vi "ReadTiffPage_next.vi"(0 "TIFF file":T2 {"BigTiff,Endian" items=["Big-Endian"=0, "Native"=1, "Little-Endian"=2, "BigTiff-Big-Endian"=256, "Bigtiff,Native"=257, "Biftiff,Littleendian"=258]}, 2 "IFDoffset":i64, 3 "error in":errorcluster) -> (6 "TIFF file out":T2 {"BigTiff,Endian" items=["Big-Endian"=0, "Native"=1, "Little-Endian"=2, "BigTiff-Big-Endian"=256, "Bigtiff,Native"=257, "Biftiff,Littleendian"=258]}, 7 "Directory Entries":T3[](array[typedef]), 9 "Next offset":i64, 10 "error out":errorcluster)   [LabVIEW 2011]
uses:
  IFD.ctl
panel:
  out "Byte-Reihenfolge (0:Big-Endian, Netzwerkreihenfolge)":T1(ring)=enum."native, host order"
  out "IFDs":u16
  # "skip read goto net IFD"
  # "seems to work!"
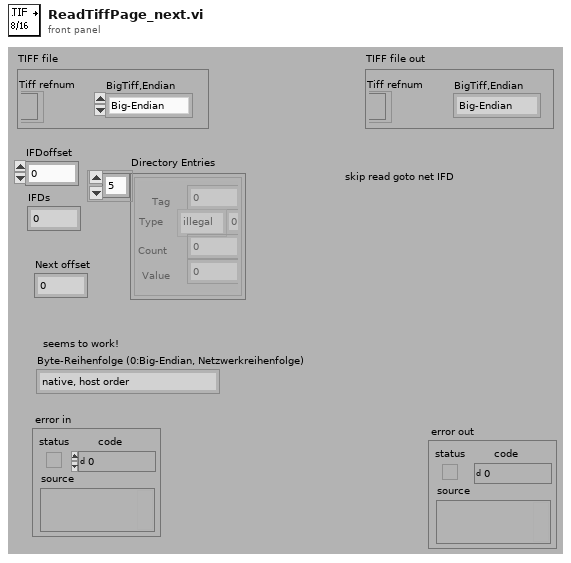
[diagram p1: front panel]
types:
  T1 = enum16{"big-endian, network order", "native, host order", "little-endian"}
  T2 = cluster{"Tiff refnum":refnum<file>, "BigTiff,Endian":u16}
  T3 = typedef "IFD.ctl" = cluster{"Tag":u16, "Type":enum16{"illegal", "Byte", "Ascii", "Short", "Long", "Rational", "SByte", "Undefined", "SShort", "SLong", "SRational 2xSLong", "Float 4byte", "Double 8Byte", "No13", "No14", "No15", "U64", "I64", "U64-IFD8"}, "Count":u64, "Value":u64}
  T4 = cluster{"Tag":u16, "Type":enum16{"illegal", "Byte", "Ascii", "Short", "Long", "Rational", "SByte", "Undefined", "SShort", "SLong", "SRational 2xSLong", "Float 4byte", "Double 8Byte"}, "Count":u32, "Value":u32}
  T5 = cluster{"Tag":u16, "Type":enum16{"illegal", "Byte", "Ascii", "Short", "Long", "Rational", "SByte", "Undefined", "SShort", "SLong", "SRational 2xSLong", "Float 4byte", "Double 8Byte"}, "Count":u32, "Value":u32}[]
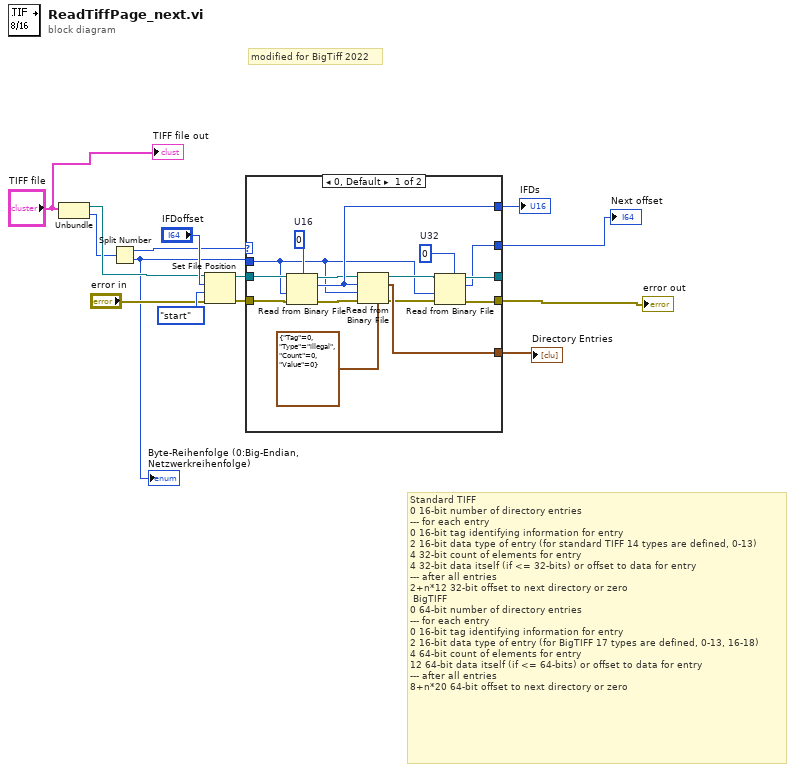
[diagram p0: block diagram]
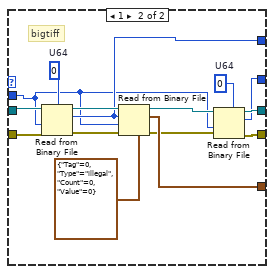
[diagram p2: hidden frame]
diagram:
  # "Standard TIFF\n0\t16-bit\tnumber of directory entries\n--- for each entry\n0\t16-bit\ttag identifying information for entry\n2\t16-bit\tdata type of entry (for standard TIFF 14 types are defined, 0-13)\n4\t32-bit\tcount of elements for entry\n4\t32-bit\tdata itself (if <= 32-bits) or offset to data for entry\n--- after all entries\n2+n*12\t32-bit\toffset to next directory or zero\n\tBigTIFF\n0\t64-bit\tnumber of directory entries\n--- for each entry\n0\t16-bit\ttag identifying information for entry\n2\t16-bit\tdata type of entry (for BigTIFF 17 types are defined, 0-13, 16-18)\n4\t64-bit\tcount of elements for entry\n12\t64-bit\tdata itself (if <= 64-bits) or offset to data for entry\n--- after all entries\n8+n*20\t64-bit\toffset to next directory or zero"
  # "modified for BigTiff 2022"
  n1 = Unbundle("TIFF file") -> ("Tiff refnum"=w10:refnum<file>, "BigTiff,Endian"=w6:u16)
  n2 = Split Number(x=w6) -> (hi(x)=w5:u8, lo(x)=w4:u8)
  "Byte-Reihenfolge (0:Big-Endian, Netzwerkreihenfolge)" <- w4
  n3 = Set File Position(offset (in bytes) (0)="IFDoffset", refnum=w10, from (0:start)=enum16{"start", "end", "current"}."start" ("pos mode (0:2)"), error in="error in") -> (refnum out=w8:refnum<file>, error out=w9:errorcluster)
  n4 = case shown="0, Default" w5 {
    tunnel: [w28 w38] -> w12
    tunnel: w9 -> [w27 w40]
    tunnel: w8 -> [w26 w39]
    tunnel: [w19 w33] -> _
    tunnel: [w18 w35] -> w1
    tunnel: [w23 w37] -> w7
    tunnel: w4 -> [w15 w32]
    tunnel: [w17 w30] -> w2
    frame 0, Default {
      w16 = u32 0  # U32
      w29 = u16 0  # U16
      n5 = Read from Binary File(5:w29, 8:w27, 9:w15, 11:w26) -> (0:w24:errorcluster, 2:w28:u16, 3:w25:refnum<file>)  [unwired: 3 out]
      n6 = Read from Binary File(5:T4 {"Tag"=0, "Type"=enum."illegal", "Count"=0, "Value"=0} ("Cluster"), 8:w24, 9:w15, 10:w28, 11:w25) -> (0:w21:errorcluster, 2:w23:T5, 3:w20:refnum<file>)  [unwired: 2 out]
      n7 = Read from Binary File(5:w16, 8:w21, 9:w15, 11:w20) -> (0:w18:errorcluster, 2:w17:u32, 3:w19:refnum<file>)  [unwired: 3 out]
    }
    frame 1 {
      w31 = u64 0  # U64
      w44 = u64 0  # U64
      # "bigtiff"
      n8 = Read from Binary File(5:w44, 8:w40, 9:w32, 11:w39) -> (0:w42:errorcluster, 2:w38:u64, 3:w43:refnum<file>)  [unwired: 3 out]
      n9 = Read from Binary File(5:T3 {"Tag"=0, "Type"=enum."illegal", "Count"=0, "Value"=0} ("Cluster"), 8:w42, 9:w32, 10:w38, 11:w43) -> (0:w36:errorcluster, 2:w37:T3[], 3:w34:refnum<file>)  [unwired: 2 out]
      n10 = Read from Binary File(5:w31, 8:w36, 9:w32, 11:w34) -> (0:w35:errorcluster, 2:w30:u64, 3:w33:refnum<file>)  [unwired: 3 out]
    }
  }
  "IFDs" <- w12
  "Directory Entries" <- w7
  "error out" <- w1
  "Next offset" <- w2
  "TIFF file out" <- "TIFF file"
